vi "D_Regulering.vi"(9 "k_d":dbl, 10 "SP":dbl, 11 "DATA":dbl) -> (2 "e(t)":dbl, 3 "u_d":dbl)   [LabVIEW 2022 SP3]
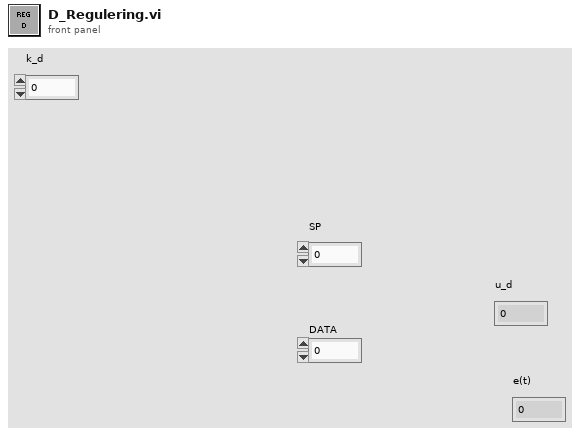
[diagram p1: front panel]
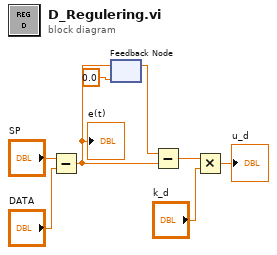
[diagram p0: block diagram]
diagram:
  n1 = Subtract(x="SP", y="DATA") -> (x-y=w1:dbl)
  "e(t)" <- w1
  n2 = feedback #1(0.0) -> (w5:dbl)
  n3 = feedback-in #1(w1) -> ()
  n4 = Subtract(x=w5, y=w1) -> (x-y=w3:dbl)
  n5 = Multiply(x=w3, y="k_d") -> (x*y=→"u_d":dbl)
